vi "校准时间.vi"() -> ()   [LabVIEW 2020]
panel:
  out "时间差":dbl
  out "计算机时间":string
  out "源表时间":string
  out "日期/时间字符串":string
  in  "校准时间":bool
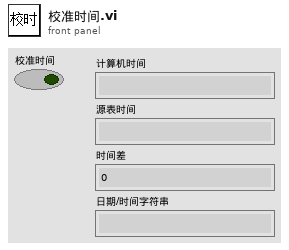
[diagram p1: front panel]
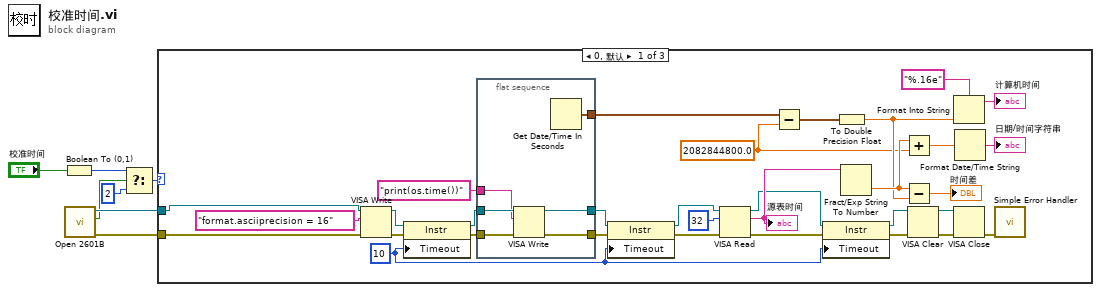
[diagram p0: block diagram]
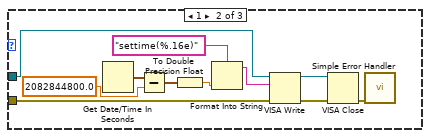
[diagram p2: hidden frame]
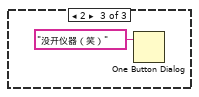
[diagram p3: hidden frame]
diagram:
  n1 = Boolean To (0,1)(Boolean="校准时间") -> (0, 1=w5:i16)
  n2 = call "Open 2601B.vi"() -> ("错误输出"=w6:errorcluster, "仪器存在"=w2:bool, "VISA资源名称输出"=w7:refnum<visa-resource-name>)  [unwired: 9 in]
  n3 = Select(t=w5, s=w2, f=i16 2) -> (s? t:f=w3:i16)
  n4 = case shown="0, 默认" w3 {
    tunnel: w6 -> [w11 w56 _]
    tunnel: w7 -> [w12 w55 _]
    frame 0, Default {
      w15 = u32 10 ("General Settings:Timeout Value")
      w16 = 2082844800.0 ("x-y")
      n5 = VISA Write(VISA resource name=w12, write buffer="format.asciiprecision = 16" ("格式字符串"), error in (no error)=w11) -> (VISA resource name out=w20:refnum<visa-resource-name>, error out=w21:errorcluster)  [unwired: 1 out]
      n6 = property class="Instr"(reference=w20, error in=w21, "Timeout"=w15) -> (reference out=w30:refnum<visa-resource-name>, error out=w31:errorcluster)
      n7 = flat-sequence {
        tunnel: [w45] -> w22
        tunnel: [w44] -> w23
        tunnel: w30 -> [w43]
        tunnel: w31 -> [w42]
        tunnel: "print(os.time())" ("写入缓冲区") -> [w41]
        tunnel: [w40] -> w33
        frame #0 {
          n8 = VISA Write(VISA resource name=w43, write buffer=w41, error in (no error)=w42) -> (VISA resource name out=w45:refnum<visa-resource-name>, error out=w44:errorcluster)  [unwired: 1 out]
          n9 = Get Date/Time In Seconds() -> (seconds since 1Jan1904=w40:timestamp)
        }
      }
      n10 = property class="Instr"(reference=w22, error in=w23, "Timeout"=w15) -> (reference out=w25:refnum<visa-resource-name>, error out=w24:errorcluster)
      n11 = VISA Read(VISA resource name=w25, byte count=u32 32 ("字节总数"), error in (no error)=w24) -> (VISA resource name out=w26:refnum<visa-resource-name>, read buffer=w32:string, error out=w27:errorcluster)  [unwired: 1 out]
      "源表时间" <- w32
      n12 = Subtract(x=w33, y=w16) -> (x-y=w34:timestamp)
      n13 = property class="Instr"(reference=w26, error in=w27, "Timeout"=w15) -> (reference out=w28:refnum<visa-resource-name>, error out=w29:errorcluster)
      n14 = To Double Precision Float(number=w34) -> (double precision float=w36:dbl)
      n15 = Fract/Exp String To Number(string=w32) -> (number=w37:dbl)  [unwired: 3 in, 1 out]
      n16 = Add(x=w37, y=w16) -> (x+y=w35:dbl)
      n17 = Subtract(x=w37, y=w36) -> (x-y=→"时间差":dbl)
      n18 = VISA Clear(VISA resource name=w28, error in (no error)=w29) -> (VISA resource name out=w8:refnum<visa-resource-name>, error out=w9:errorcluster)
      n19 = Format Into String(format string="%.16e" ("格式字符串"), w36) -> (resulting string=→"计算机时间":string)  [unwired: 2 in, 1 out]
      n20 = VISA Close(VISA resource name=w8, error in (no error)=w9) -> (error out=w10:errorcluster)
      n21 = Format Date/Time String(seconds (now)=w35) -> (date/time string=→"日期/时间字符串":string)  [unwired: 2 in]
      n22 = call <vilib>:"Simple Error Handler.vi"("error in (no error)"=w10) -> ()  [unwired: 4 in, 5 out]
    }
    frame 1 {
      n23 = Get Date/Time In Seconds() -> (seconds since 1Jan1904=w52:timestamp)
      n24 = Subtract(x=w52, y=2082844800.0 ("x-y")) -> (x-y=w53:timestamp)
      n25 = To Double Precision Float(number=w53) -> (double precision float=w54:dbl)
      n26 = Format Into String(format string="settime(%.16e)" ("格式字符串"), w54) -> (resulting string=w49:string)  [unwired: 2 in, 1 out]
      n27 = VISA Write(VISA resource name=w55, write buffer=w49, error in (no error)=w56) -> (VISA resource name out=w47:refnum<visa-resource-name>, error out=w46:errorcluster)  [unwired: 1 out]
      n28 = VISA Close(VISA resource name=w47, error in (no error)=w46) -> (error out=w48:errorcluster)
      n29 = call <vilib>:"Simple Error Handler.vi"("error in (no error)"=w48) -> ()  [unwired: 4 in, 5 out]
    }
    frame 2 {
      n30 = One Button Dialog(message="没开仪器（笑）" ("消息")) -> ()  [unwired: 1 in, 1 out]
    }
  }
